vi "ParseStateQueue.vi"(0 "State Queue":string, 1 "MemoryStateSize(25)":i32=25, 7 "Error In (no error)":errorcluster) -> (2 "StatePlusArgument(ForLogging)":string, 3 "Previous State with Arguments":string, 4 "Remaining States":string, 6 "Current State":string, 8 "Arguments":string)   [LabVIEW 2020]
doc: "Parses the State Machine state queue and returns the current state that will execute next with the associated arguments.\n\n<B>Inputs:</B>\n <B>State Queue:</B> The entire state queue is wired to this input. \n <B>Error In</B> The error cluster from the State Machine is wired to this input. If an error occures and appears on this input, the current state output returns the \"Error Handler\" state.\n\n<B>Outputs:</B>\n <B>Remaining States:</B> Returns all the next states that should execute after the current state completes. These should be passed through the current state in the state machine. These can also be modified or augmented within the current state if necessary.\n <B>Current State:</B> Returns the current state that should execute next in the state machine. If an error is wired to the Error input then the current state output becomes \"Error Handler\".\n <B>Arguments:</B> Returns any argument(s) that may be used in the current state string. These arguments come after the \">>\" characters. <B>Note:</B> The arguments variable must not contain any unprintable characters like linefeed or carriage return.\n <B>Previous State:</B> Returns the previous state that was execute last in the state machine.\n\n<B>State Syntax:</B>\nStateCategory: State >> Argument\nLine Terminator: Line feed\n <B>Example:</B>\nUI: Help >> About\n\nWhere \"UI\" is the state category\nWhere \"Help\" is the state\nWhere \"About\" is the argument\n <B>Other Examples:</B>\nApp Data: Initialize\nUI: Initialize\nHelp >> About\n\n<B>Commenting:</B>\nTo add a comment use \"//\" or \"#\" and all text to the right will be ignored\n <B>Commenting Example:</B>\nUI: Initialize // This initializes the UI\n# This whole line is a comment\n// Another comment line"
panel:
  # "For instructions on how to use the JKI State Machine, examples and video tutorials, visit:\nhttp://jkisoft.com/state-machine/\n\nJKI State Machine™\nhttp://jkisoft.com/state-machine/\nCopyright (C) 2005-2008, JKI <info@jkisoft.com>\nALL RIGHTS RESERVED"
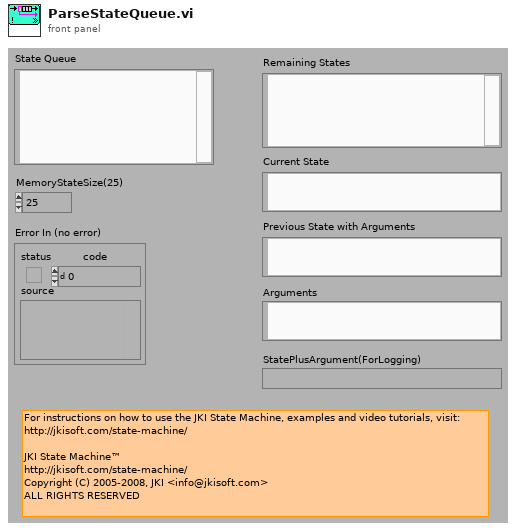
[diagram p1: front panel]
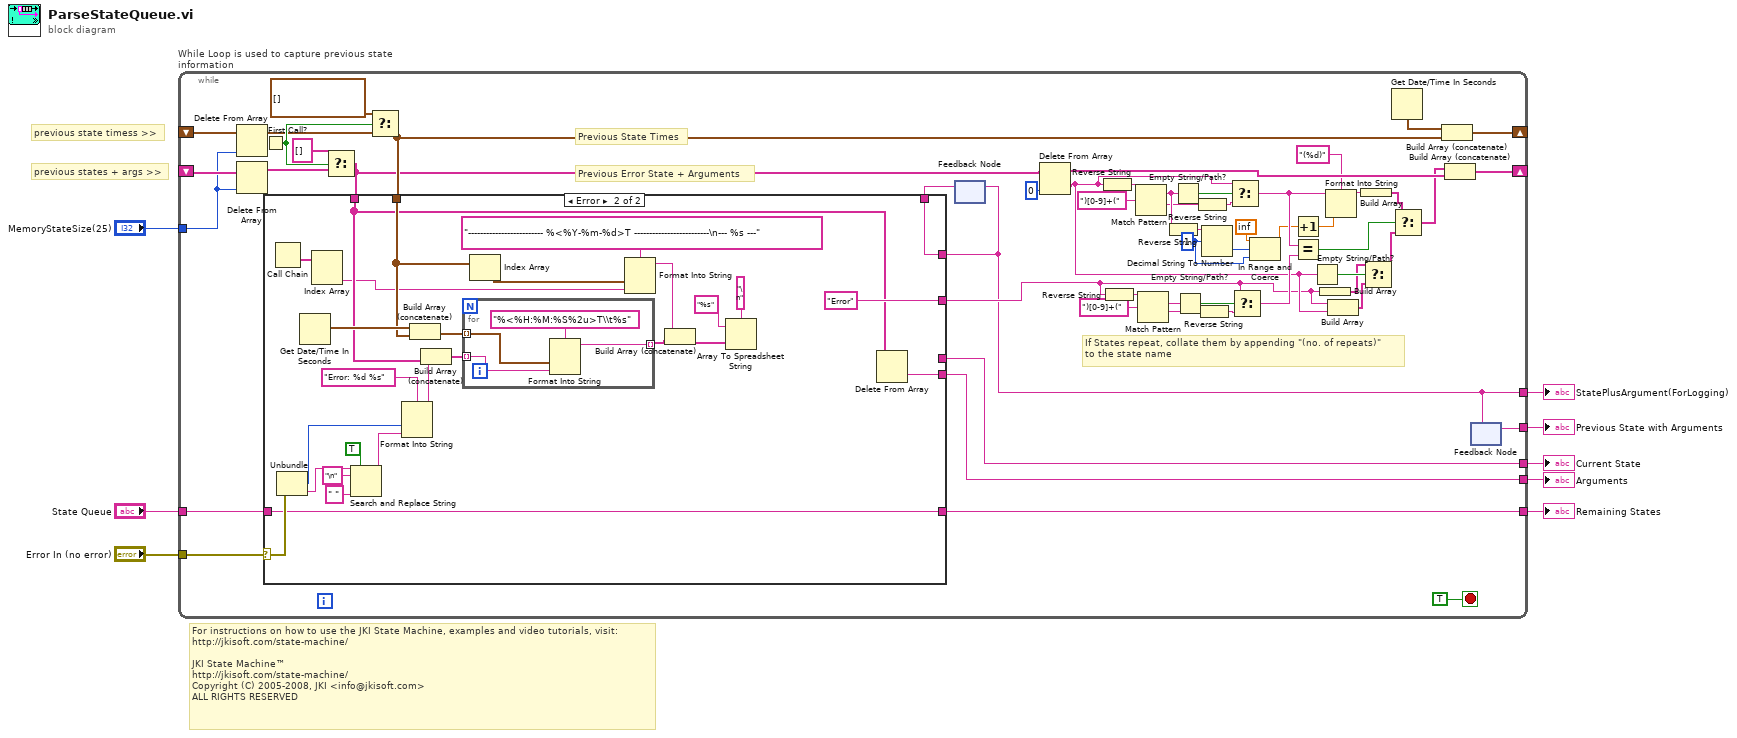
[diagram p0: block diagram]
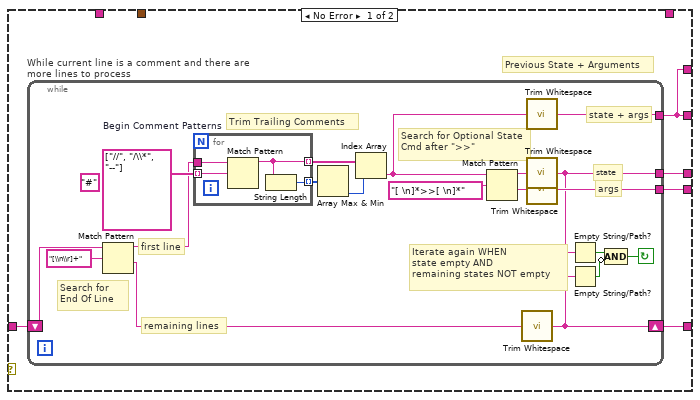
[diagram p2: hidden frame]
diagram:
  # "For instructions on how to use the JKI State Machine, examples and video tutorials, visit:\nhttp://jkisoft.com/state-machine/\n\nJKI State Machine™\nhttp://jkisoft.com/state-machine/\nCopyright (C) 2005-2008, JKI <info@jkisoft.com>\nALL RIGHTS RESERVED"
  # "previous state timess >>"
  # "previous states + args >>"
  n1 = while "While Loop is used to capture previous state information" {
    tunnel: [w62] -> w7
    tunnel: "State Queue" -> [w61]
    tunnel: "Error In (no error)" -> [w63]
    tunnel: [w11] -> w5
    tunnel: [w60] -> w4
    shift-right: [w15] -> _
    shift-left: _ -> [w51]
    shift-right: [w57] -> _
    shift-left: _ -> [w53]
    tunnel: "MemoryStateSize(25)" -> [w14]
    tunnel: [w9] -> w2
    tunnel: [w10] -> w1
    stop <- TRUE stop-if-true
    w24 = 1 ("offset")
    # "If States repeat, collate them by appending \"(no. of repeats)\"\nto the state name"
    # "Previous State Times"
    # "Previous Error State + Arguments"
    n2 = Delete From Array(array=w53, index=w14) -> (array with subset deleted=w52:timestamp[])  [unwired: 1 in, 1 out]
    n3 = Delete From Array(array=w51, index=w14) -> (array with subset deleted=w50:string[])  [unwired: 1 in, 1 out]
    n4 = First Call?() -> (First Call?: T/F=w55:bool)
    n5 = Select(t=string[] [], s=w55, f=w50) -> (s? t:f=w48:string[])
    n6 = Select(t=timestamp[] [], s=w55, f=w52) -> (s? t:f=w49:timestamp[])
    n7 = feedback #1() -> (w12:string)  [unwired: 1 in]
    n8 = case shown="Error" w63 {
      selector: w63 -> [_ w118]
      tunnel: [w65 w117] -> w62
      tunnel: [w68 w116] -> w11
      tunnel: [w67 w115] -> w60
      tunnel: w61 -> [w66 w117]
      tunnel: [w64 w116] -> w13
      tunnel: w48 -> [_ w104]
      tunnel: w49 -> [_ w106]
      tunnel: [w64 w95] -> w9
      tunnel: w12 -> [_ w95]
      frame No Error {
        # "Previous State + Arguments"
        n9 = while "While current line is a comment and there are more lines to process" {
          tunnel: [w78] -> w68
          tunnel: [w79] -> w67
          shift-right: [w74] -> w65
          shift-left: w66 -> [w72]
          tunnel: [w69] -> w64
          stop <- w75 continue-if-true
          (unwired) "#"
          w86 = string[] ["//", "/\\*", "--"]  # Begin Comment Patterns
          # "state + args"
          # "remaining lines"
          # "first line"
          # "Search for End Of Line"
          # "Iterate again WHEN\nstate empty AND\nremaining states NOT empty"
          # "args"
          # "state"
          # "Search for Optional State Cmd after \">>\""
          # "Trim Trailing Comments"
          n10 = Match Pattern(string=w72, regular expression="[\\n\\r]+") -> (before substring=w71:string, after substring=w87:string)  [unwired: 3 out]
          n11 = for {
            tunnel: w71 -> [w91]
            tunnel: [w89] -> w83 mode=indexing
            tunnel: w86 -> [w90] mode=indexing
            tunnel: [w88] -> w85 mode=indexing
            n12 = Match Pattern(string=w91, regular expression=w90) -> (before substring=w89:string)  [unwired: 4 out]
            n13 = String Length(string=w89) -> (length=w88:i32)
          }
          n14 = Array Max & Min(array=w85) -> (min index (indices)=w84:i32)  [unwired: 3 out]
          n15 = Index Array(array=w83, index=w84) -> (element=w70:string)
          n16 = Match Pattern(string=w70, regular expression="[ \n]*>>[ \n]*") -> (before substring=w81:string, after substring=w80:string)  [unwired: 3 out]
          n17 = call <vilib>:"Trim Whitespace.vi"("string"=w87) -> ("trimmed string"=w74:string)  [unwired: 1 in]
          n18 = call <vilib>:"Trim Whitespace.vi"("string"=w70) -> ("trimmed string"=w69:string)  [unwired: 1 in]
          n19 = call <vilib>:"Trim Whitespace.vi"("string"=w81) -> ("trimmed string"=w78:string)  [unwired: 1 in]
          n20 = call <vilib>:"Trim Whitespace.vi"("string"=w80) -> ("trimmed string"=w79:string)  [unwired: 1 in]
          n21 = Empty String/Path?(string/path=w78) -> (empty?=w77:bool)
          n22 = Empty String/Path?(string/path=w74) -> (empty?=w76:bool)
          n23 = Compound Arithmetic op=AND(w77, invert w76) -> (w75:bool)
        }
      }
      frame Error {
        w116 = "Error"
        n24 = Call Chain() -> (call chain=w94:string[])
        n25 = Unbundle(w118) -> ("code"=w92:i32, "source"=w101:string)  [unwired: 1 out]
        n26 = Get Date/Time In Seconds() -> (seconds since 1Jan1904=w107:timestamp)
        n27 = Index Array(array=w94) -> (element #2=w93:string)  [unwired: 2 in, 1 out]
        n28 = Search and Replace String(replace all?=TRUE ("replace all? (F)"), input string=w101, search string="\n", replace string=" " ("replace string (\"\")")) -> (result string=w96:string)  [unwired: 1 in, 6 out]
        n29 = Format Into String(format string="Error: %d %s", w92, w96) -> (resulting string=w97:string)  [unwired: 2 in, 1 out]
        n30 = Build Array (concatenate)(w107, w106) -> (w105:timestamp[])
        n31 = Build Array (concatenate)(w97, w104) -> (w103:string[])
        n32 = for {
          tunnel: w103 -> [w120] mode=indexing
          tunnel: w105 -> [w121] mode=indexing
          tunnel: [w119] -> w109 mode=indexing
          n33 = Format Into String(format string="%<%H:%M:%S%2u>T\\t%s", w121, w120) -> (resulting string=w119:string)  [unwired: 2 in, 1 out]
        }
        n34 = Index Array(array=w106) -> (element=w111:timestamp)  [unwired: 1 in]
        n35 = Format Into String(format string="------------------------- %<%Y-%m-%d>T -------------------------\n--- %s ---", w111, w93) -> (resulting string=w110:string)  [unwired: 2 in, 1 out]
        n36 = Build Array (concatenate)(w110, w109) -> (w108:string[])
        n37 = Array To Spreadsheet String(delimiter (Tab)="\n", array=w108, 3:"%s" ("format string")) -> ()  [unwired: 1 out]
        n38 = Delete From Array(array=w104) -> (deleted portion=w115:string)  [unwired: 2 in, 1 out]
      }
    }
    n39 = feedback-in #1(w9) -> ()
    n40 = Delete From Array(array=w48, index=0) -> (deleted portion=w19:string, array with subset deleted=w32:string[])  [unwired: 1 in]
    n41 = Reverse String(1:w19) -> (0:w47:string)
    n42 = Reverse String(1:w13) -> (0:w35:string)
    n43 = Match Pattern(string=w47, regular expression=")[0-9]+(") -> (match substring=w45:string, after substring=w43:string)  [unwired: 1 in, 2 out]
    n44 = Match Pattern(string=w35, regular expression=")[0-9]+(") -> (match substring=w37:string, after substring=w39:string)  [unwired: 1 in, 2 out]
    n45 = Reverse String(1:w45) -> (0:w41:string)
    n46 = Empty String/Path?(string/path=w45) -> (empty?=w44:bool)
    n47 = Empty String/Path?(string/path=w37) -> (empty?=w38:bool)
    n48 = Reverse String(1:w43) -> (0:w42:string)
    n49 = Reverse String(1:w39) -> (0:w40:string)
    n50 = Decimal String To Number(string=w41, offset=w24) -> (number=w25:i32)  [unwired: 1 in, 1 out]
    n51 = Select(t=w19, s=w44, f=w42) -> (s? t:f=w30:string)
    n52 = Select(t=w13, s=w38, f=w40) -> (s? t:f=w34:string)
    n53 = In Range and Coerce(upper limit=inf, x=w25, lower limit=w24) -> (coerced(x)=w22:dbl)  [unwired: 1 out]
    n54 = Increment(x=w22) -> (x+1=w29:dbl)
    n55 = Equal?(x=w30, y=w34) -> (x = y?=w21:bool)
    n56 = Empty String/Path?(string/path=w19) -> (empty?=w20:bool)
    n57 = Build Array(w13) -> (w16:string[])
    n58 = Format Into String(format string="(%d)" ("regular expression"), initial string=w30, w29) -> (resulting string=w27:string)  [unwired: 1 in, 1 out]
    n59 = Build Array(w13, w19) -> (w17:string[])
    n60 = Build Array(w27) -> (w26:string[])
    n61 = Select(t=w16, s=w20, f=w17) -> (s? t:f=w18:string[])
    n62 = Get Date/Time In Seconds() -> (seconds since 1Jan1904=w56:timestamp)
    n63 = Select(t=w26, s=w21, f=w18) -> (s? t:f=w31:string[])
    n64 = Build Array (concatenate)(w56, w49) -> (w57:timestamp[])
    n65 = Build Array (concatenate)(w31, w32) -> (w15:string[])
    n66 = feedback-in #2(w9) -> ()
    n67 = feedback #2() -> (w10:string)  [unwired: 1 in]
  }
  "Remaining States" <- w7
  "Arguments" <- w4
  "Current State" <- w5
  "StatePlusArgument(ForLogging)" <- w2
  "Previous State with Arguments" <- w1
